vi "AddModule.vi"(5 "module":T1, 6 "error in":errorcluster, 9 "PythonConverter_GUI in":refnum<class "PythonConverter_GUI.lvclass">) -> (0 "error out":errorcluster, 3 "PythonConverter_GUI out":refnum<class "PythonConverter_GUI.lvclass">)   [LabVIEW 2014, in "Raspberry Pi Compatible Compiler for LabVIEW.lvlib" / "PythonConverter_GUI.lvclass"]
uses:
  PythonConverter_GUI.lvclass
  TypeDefs/PythonModuleTD.ctl
  PythonConverter_GUI.lvclass/PythonConverter_GUI.ctl
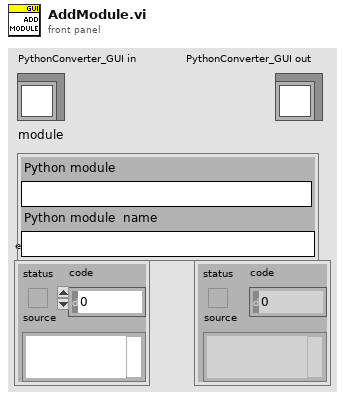
[diagram p1: front panel]
types:
  T1 = typedef "Raspberry Pi Compatible Compiler for LabVIEW.lvlib/PythonConverter_GUI.lvclass/PythonModuleTD.ctl" = cluster{"Python module":string, "Python module  name":string}
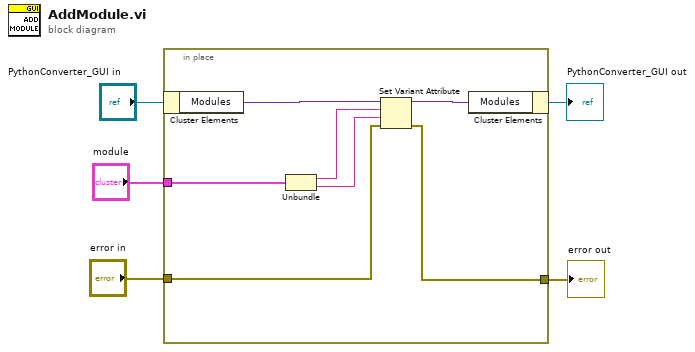
[diagram p0: block diagram]
diagram:
  n1 = in-place {
    in-place-border: "error in" -> [w10]
    in-place-border: [w9] -> w2
    in-place-border: "module" -> [w8]
    n2 = in-place-cluster #1("PythonConverter_GUI in") -> ("Modules"=w12:variant)
    n3 = Unbundle(w8) -> ("Python module"=w7:string, "Python module  name"=w6:string)
    n4 = Set Variant Attribute(Variant=w12, name=w7, value=w6, error in=w10) -> (Variant out=w11:variant, error out=w9:errorcluster)  [unwired: 1 out]
    n5 = in-place-cluster #1("Modules"=w11) -> (→"PythonConverter_GUI out":refnum<class "PythonConverter_GUI.lvclass">)
  }
  "error out" <- w2
